vi "intensityGraph.vi"() -> ()   [LabVIEW 2014]
panel:
  in  "Scale Factor":dbl(slide) scale=0.0..10.0
  out "Intensity Graph":dbl[][](graph)
  in  "Number of Row/Columns":i32(slide) scale=0.0..100.0
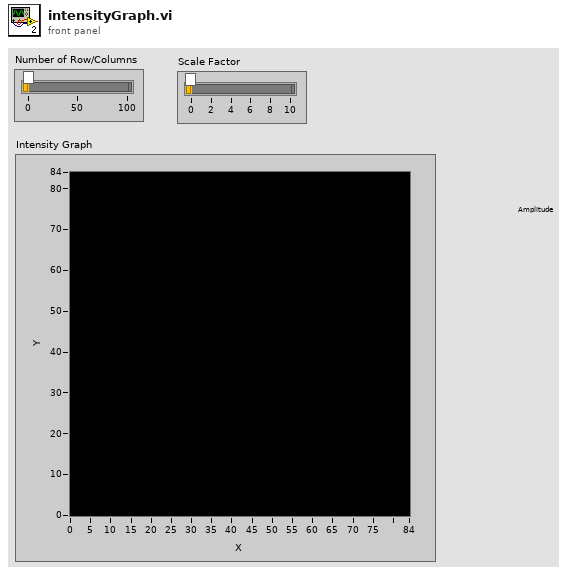
[diagram p1: front panel]
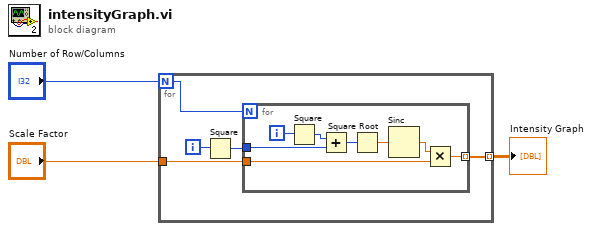
[diagram p0: block diagram]
diagram:
  n1 = for {
    N: "Number of Row/Columns" -> [w5]
    tunnel: [w6] -> w2 mode=indexing
    tunnel: "Scale Factor" -> [w4]
    i -> [w8]
    n2 = Square(x=w8) -> (x^2=w7:i32)
    n3 = for {
      N: w5 -> [_]
      tunnel: w7 -> [w14]
      tunnel: [w10] -> w6 mode=indexing
      tunnel: w4 -> [w9]
      i -> [w16]
      n4 = Square(x=w16) -> (x^2=w13:i32)
      n5 = Add(x=w13, y=w14) -> (x+y=w15:i32)
      n6 = Square Root(x=w15) -> (sqrt(x)=w12:dbl)
      n7 = Sinc(1:w12) -> (0:w11:dbl)
      n8 = Multiply(x=w11, y=w9) -> (x*y=w10:dbl)
    }
  }
  "Intensity Graph" <- w2
